vi "What Type Pos Correct.vi"(9 "Point Out":cluster{dbl, dbl}, 10 "Array":T1(array[cluster])) -> (3 "Cluster out":T2)   [LabVIEW 2025]
uses:
  <vilib>/vision/NI_Vision_Development_Module.lvlib
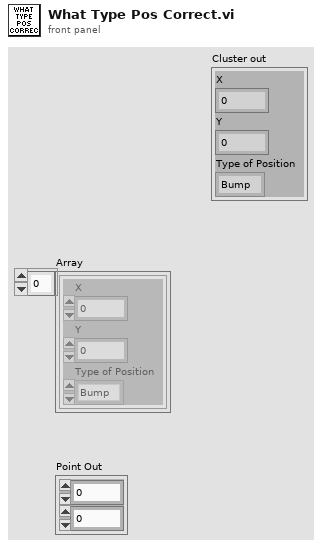
[diagram p1: front panel]
types:
  T1 = cluster{"X":dbl, "Y":dbl, "Type of Position":enum16{"Bump", "Close Shooter Shot"}}[]
  T2 = cluster{"X":dbl, "Y":dbl, "Type of Position":enum16{"Bump", "Close Shooter Shot"}}
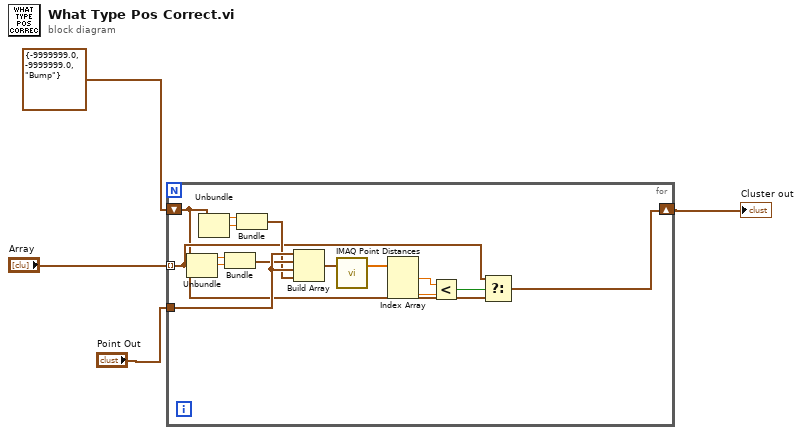
[diagram p0: block diagram]
diagram:
  n1 = for {
    tunnel: "Array" -> [w7] mode=indexing
    tunnel: "Point Out" -> [w15]
    shift-right: [w5] -> w4
    shift-left: T2 {"X"=-9999999.0, "Y"=-9999999.0, "Type of Position"=enum."Bump"} ("Cluster") -> [w6]
    n2 = Unbundle(w7) -> ("X"=w19:dbl, "Y"=w18:dbl)  [unwired: 1 out]
    n3 = Unbundle(w6) -> ("X"=w17:dbl, "Y"=w16:dbl)  [unwired: 1 out]
    n4 = Bundle("X"=w19, "Y"=w18) -> (w14:cluster{"X":dbl, "Y":dbl})  [unwired: 1 in]
    n5 = Bundle("X"=w17, "Y"=w16) -> (w13:cluster{"X":dbl, "Y":dbl})  [unwired: 1 in]
    n6 = Build Array(w15, w14, w15, w13) -> (w12:cluster{"X":dbl, "Y":dbl}[])
    n7 = call "IMAQ Point Distances"("Points"=w12) -> ("Distances"=w11:sgl[])  [unwired: 4 in, 1 out]
    n8 = Index Array(array=w11) -> (element #1=w10:sgl, element #3=w9:sgl)  [unwired: 3 in, 1 out]
    n9 = Less?(x=w10, y=w9) -> (x < y?=w8:bool)
    n10 = Select(t=w7, s=w8, f=w6) -> (s? t:f=w5:T2)
  }
  "Cluster out" <- w4
